vi "_084.vi"() -> ()   [LabVIEW 2024]
panel:
  out "min index(es) 2":i32[](array[numeric])
  out "min value 2":i32
  out "max index(es) 2":i32[](array[numeric])
  out "max value 4":i32
  out "subarray":i32[][](array[numeric])
  out "Array 3":dbl[][](array[numeric])
  out "Array 2":dbl[][](array[numeric])
  out "max value 3":i32
  out "Array":dbl[][](array[numeric])
  out "max value 2":i32
  out "min index(es)":i32[](array[numeric])
  out "min value":i32
  out "max index(es)":i32[](array[numeric])
  out "max value":i32
  # "Fundamentals :"
  # "13~>After running this VI,what is the value displayed in the o/p ?"
  # "Nrml Approach :"
  # "Dfrnt Approach :"
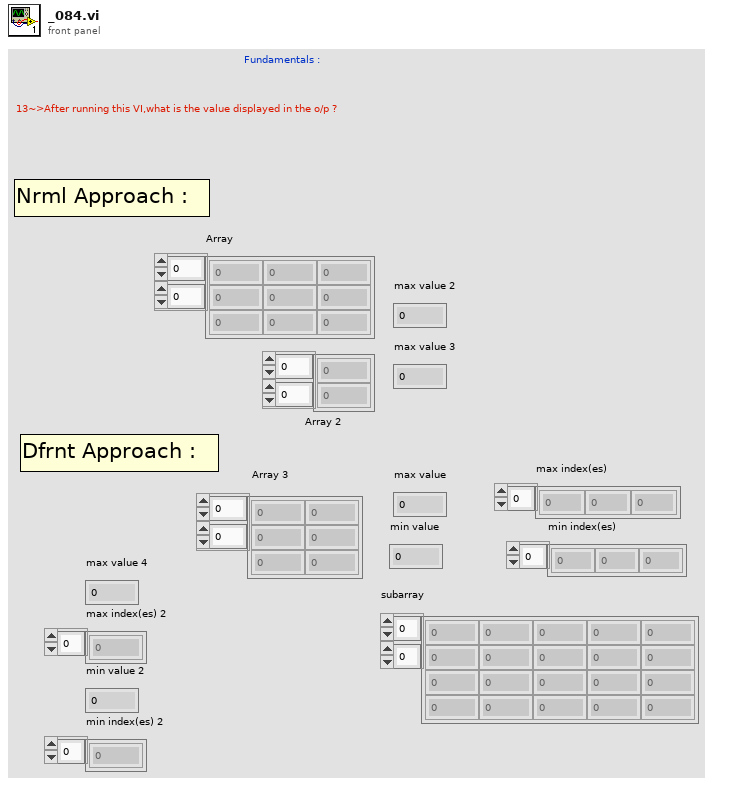
[diagram p1: front panel]
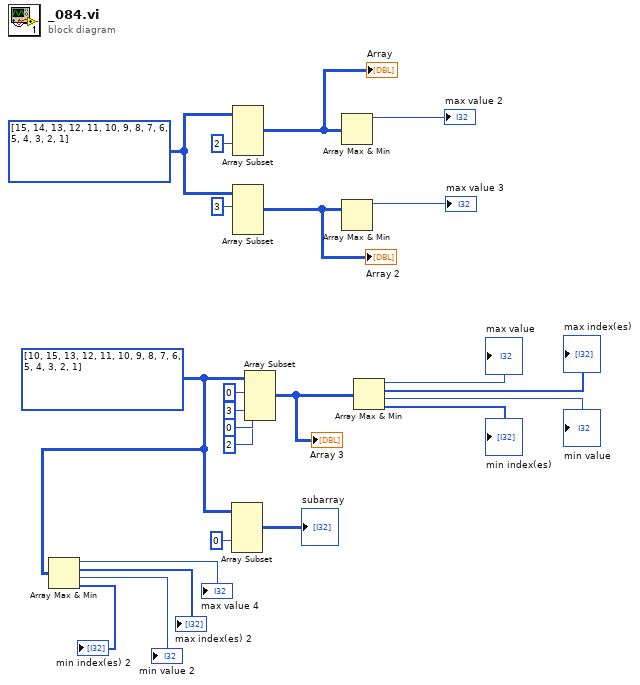
[diagram p0: block diagram]
diagram:
  w12 = i32[][] [[15, 14, 13, 12, 11], [10, 9, 8, 7, 6], [5, 4, 3, 2, 1]]
  w5 = i32[][] [[10, 15, 13, 12, 11], [10, 9, 8, 7, 6], [5, 4, 3, 2, 1]]
  n1 = Array Max & Min(array=w5) -> (max value=→"max value 4":i32, max index (indices)=→"max index(es) 2":i32[], min value=→"min value 2":i32, min index (indices)=→"min index(es) 2":i32[])
  n2 = Array Subset "Array Subset"(array=w5, index (col)=0 ("index")) -> (→"subarray":i32[][])  [unwired: 3 in]
  n3 = Array Subset "Array Subset"(array=w12, index (col)=2 ("index")) -> (w13:i32[][])  [unwired: 3 in]
  "Array" <- w13
  n4 = Array Subset "Array Subset"(array=w12, index (row)=3 ("index")) -> (w9:i32[][])  [unwired: 3 in]
  "Array 2" <- w9
  n5 = Array Subset "Array Subset"(array=w5, index (row)=0 ("index"), length (row)=3 ("length"), index (col)=0 ("index"), length (col)=2 ("length")) -> (w8:i32[][])
  "Array 3" <- w8
  n6 = Array Max & Min(array=w13) -> (max value=→"max value 2":i32)  [unwired: 3 out]
  n7 = Array Max & Min(array=w9) -> (max value=→"max value 3":i32)  [unwired: 3 out]
  n8 = Array Max & Min(array=w8) -> (max value=→"max value":i32, max index (indices)=→"max index(es)":i32[], min value=→"min value":i32, min index (indices)=→"min index(es)":i32[])
